vi "Write DAC On.vi"(8 "error in (no error)":errorcluster, 10 "DAC On":bool, 11 "DAC in":refnum<class "DAC.lvclass">) -> (0 "error out":errorcluster, 3 "DAC out":refnum<class "DAC.lvclass">)   [LabVIEW 2019, in "DAC.lvlib" / "DAC.lvclass"]
uses:
  DAC.lvclass
  DAC.lvclass/DAC.ctl
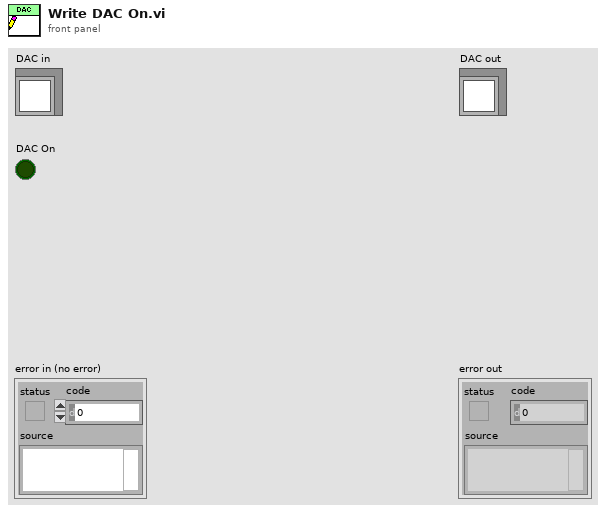
[diagram p1: front panel]
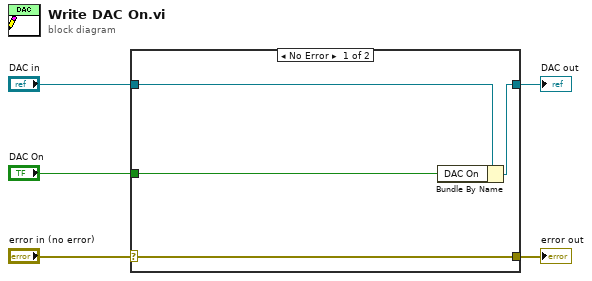
[diagram p0: block diagram]
diagram:
  n1 = case shown="No Error" "error in (no error)" {
    selector: "error in (no error)" -> [w9 w10]
    tunnel: [w9 w10] -> w4
    tunnel: [w7 w11] -> w2
    tunnel: "DAC in" -> [w8 w11]
    tunnel: "DAC On" -> [w6 _]
    frame No Error {
      n2 = Bundle By Name(cluster=w8, "DAC On"=w6) -> (w7:refnum<class "DAC.lvclass">)
    }
    frame Error {
    }
  }
  "error out" <- w4
  "DAC out" <- w2
